vi "Config Save As.vi"(0 "Config Dir":path=path "C:/Users/gtetil/Documents/Projects/TI-cDAQ/Source/Support/Configurations", 1 "Config Extension":string="*.std", 2 "Config Name":string="test.std", 5 "Error IN":errorcluster) -> (14 "Save As":bool, 15 "Config Name OUT":string, 19 "Error OUT":errorcluster)   [LabVIEW 2023]
panel:
  out "Extension":string
  in  "New Config Name:":string caption="Config Name:"
  in  "Cancel Button":bool
  in  "Save As":bool
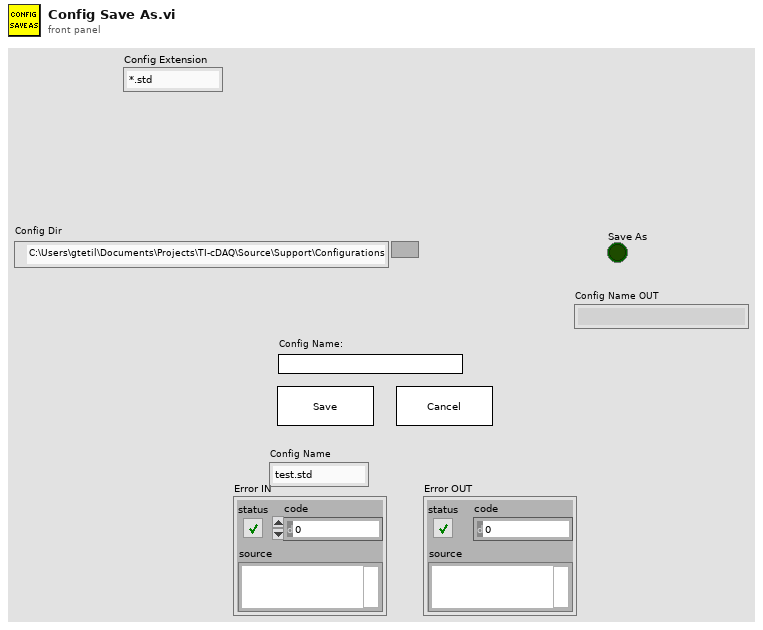
[diagram p1: front panel]
types:
  T1 = cluster{"Error IN":errorcluster, "Config Dir":path, "Config Extension":string, "Save As":bool, "Config Name":string, "Config List":string[]}
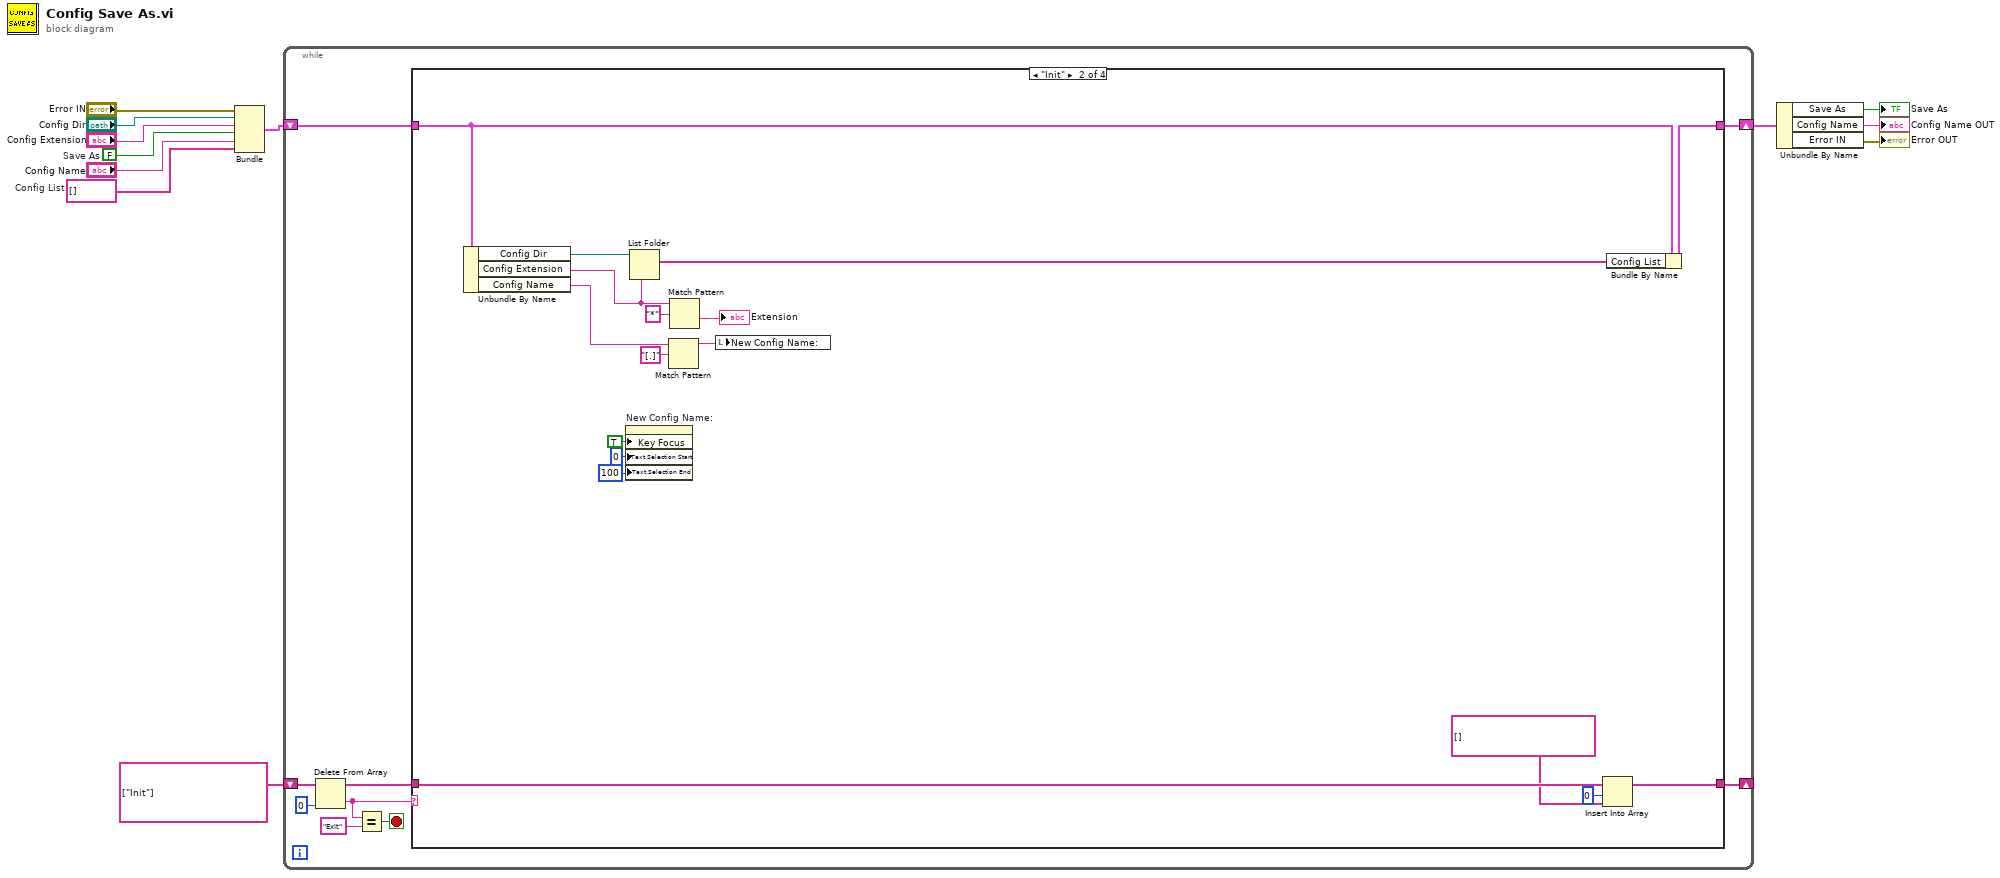
[diagram p0: block diagram]
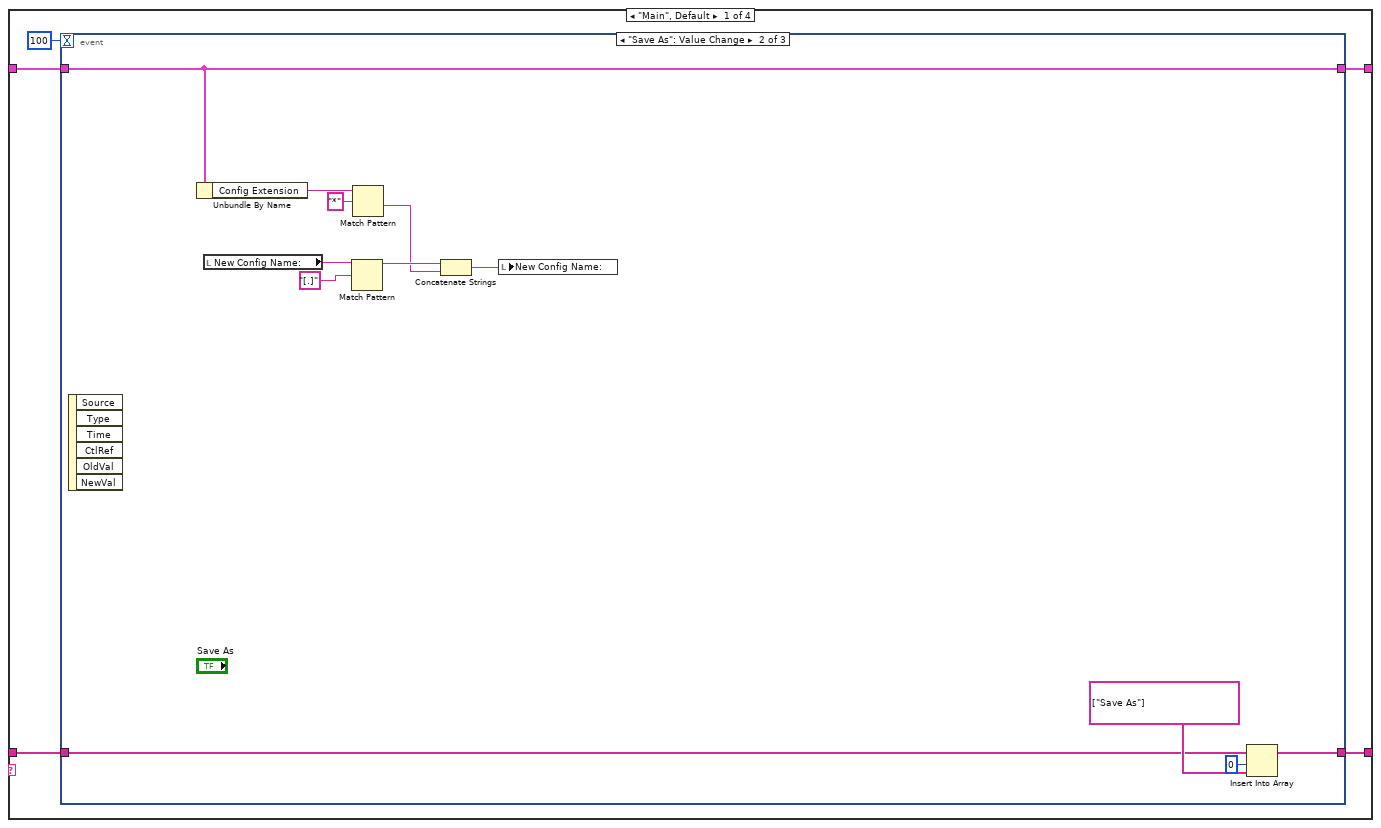
[diagram p2: hidden frame]
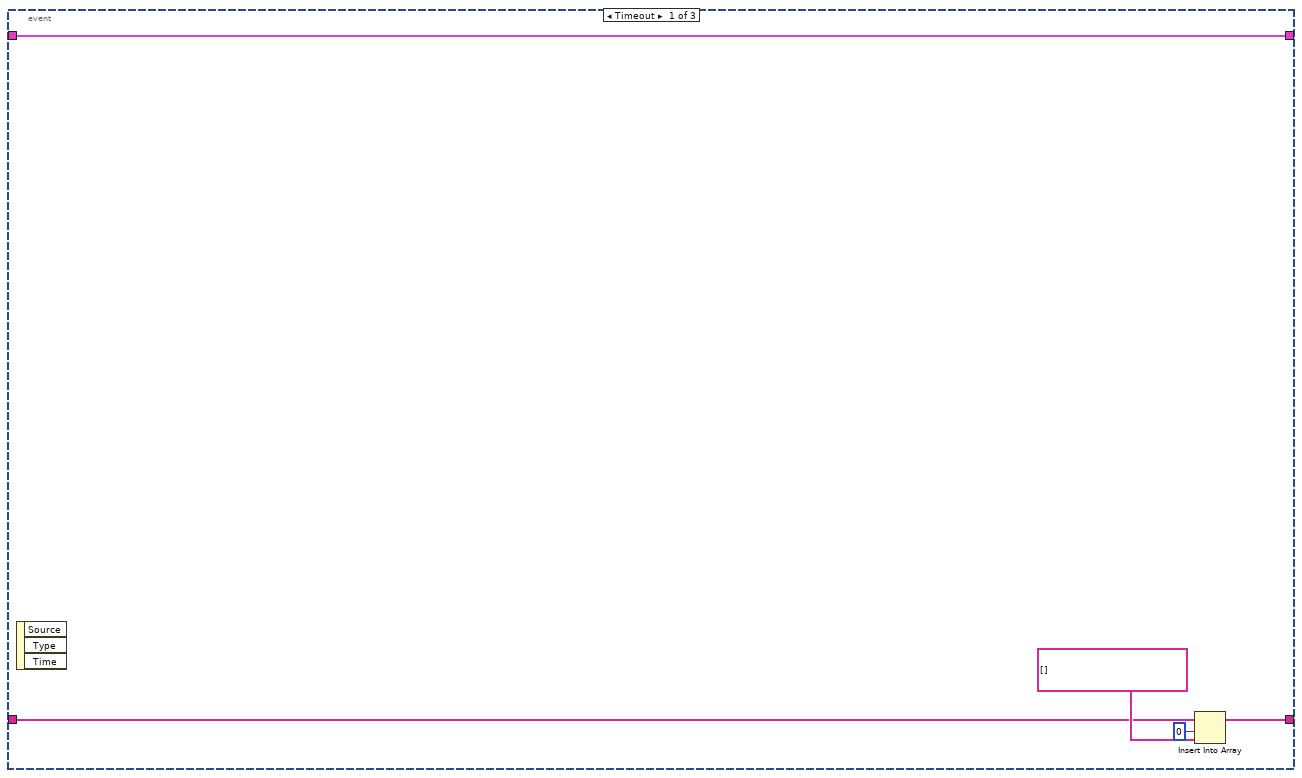
[diagram p3: hidden frame]
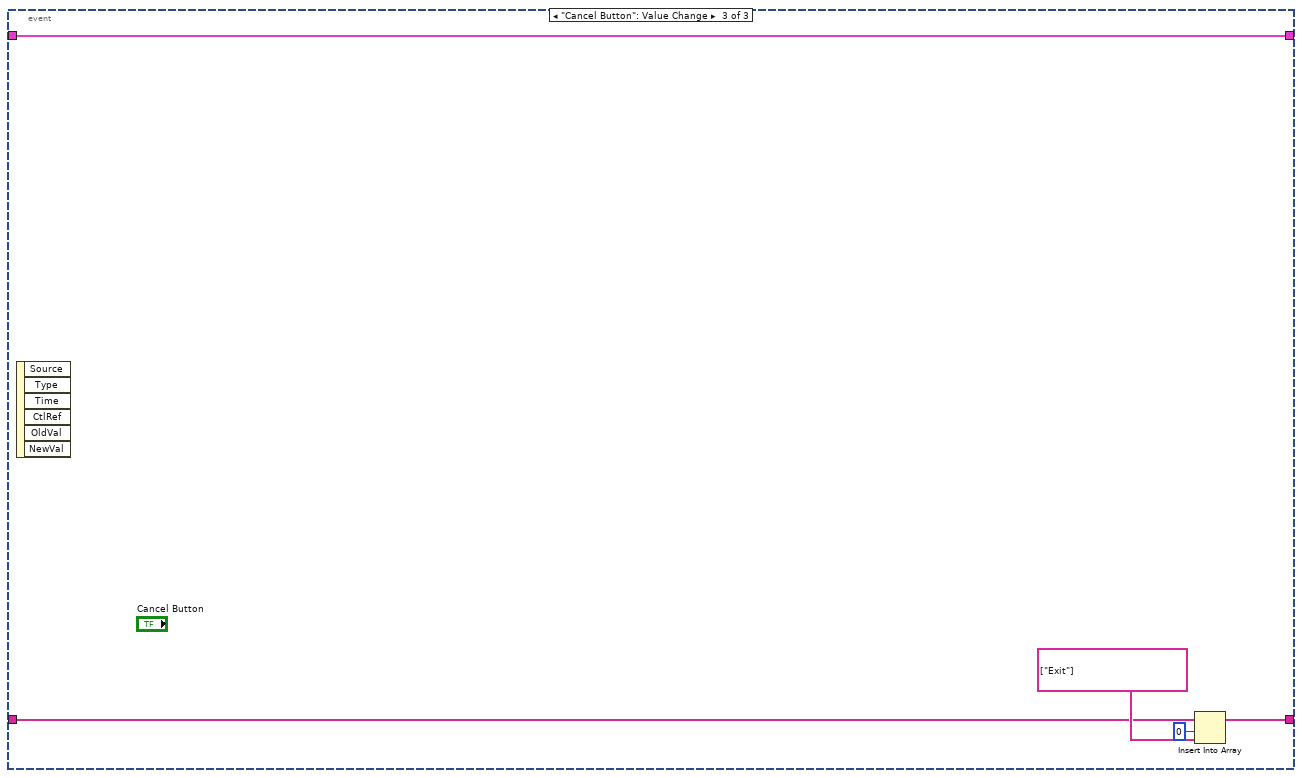
[diagram p4: hidden frame]
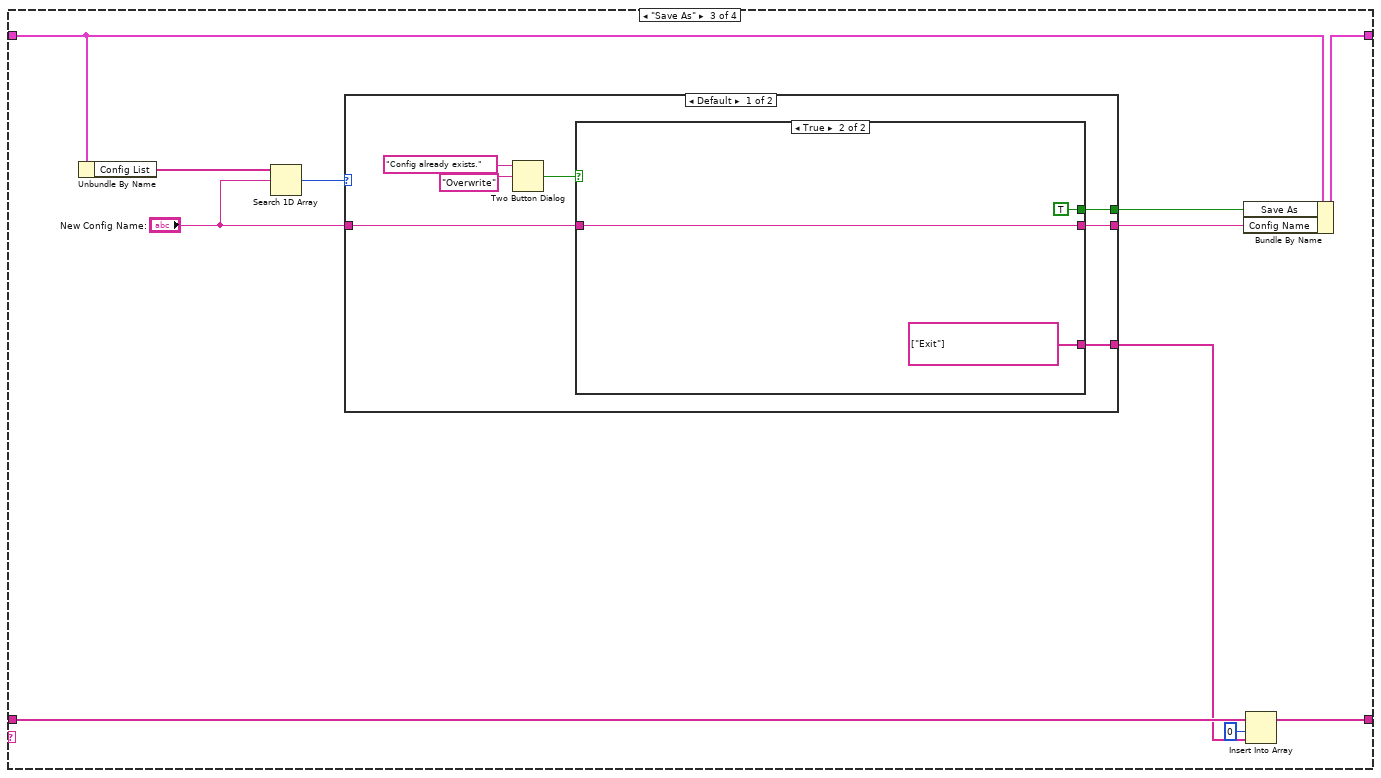
[diagram p5: hidden frame]
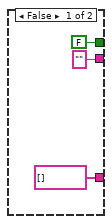
[diagram p6: hidden frame]
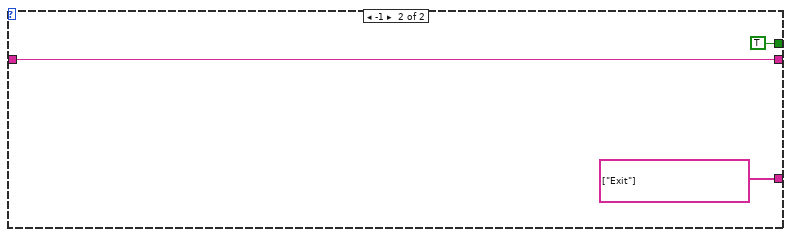
[diagram p7: hidden frame]
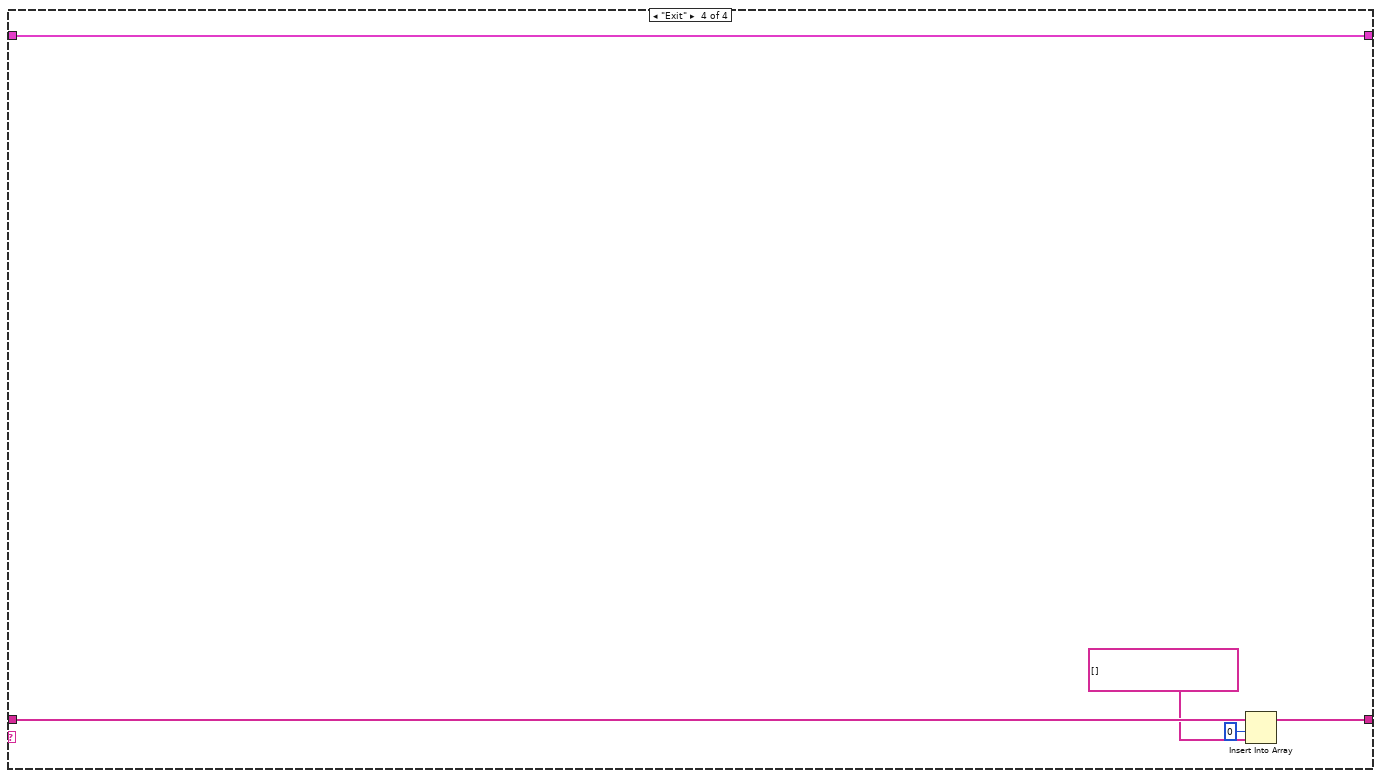
[diagram p8: hidden frame]
diagram:
  w2 = string[] []  # Config List
  w4 = FALSE  # Save As
  n1 = Bundle("Error IN"="Error IN", "Config Dir"="Config Dir", "Config Extension"="Config Extension", "Save As"=w4, "Config Name"="Config Name", "Config List"=w2) -> (w6:T1)  [unwired: 1 in]
  n2 = while {
    shift-right: [w16] -> _
    shift-left: string[] ["Init"] -> [w21]
    shift-right: [w13] -> w9
    shift-left: w6 -> [w14]
    stop <- w17 stop-if-true
    n3 = Delete From Array(array=w21, index=0 ("length")) -> (deleted portion=w18:string, array with subset deleted=w15:string[])  [unwired: 1 in]
    n4 = Equal?(x=w18, y="Exit") -> (x = y?=w17:bool)
    n5 = case shown="\"Init\"" w18 {
      tunnel: [w22 w65 w76 w97] -> w16
      tunnel: w15 -> [w23 w64 w75 w96]
      tunnel: w14 -> [w26 w59 w72 w93]
      tunnel: [w25 w60 w73 w93] -> w13
      frame "Main", Default {
        n6 = event shown="[1] \"Save As\": Value Change" {
          selector: _ -> [_ _ _]
          dyn-events: _ -> [_ _ _]
          timeout: 100 -> [_ _ _]
          tunnel: w26 -> [w31 w39 w44]
          tunnel: [w31 w39 w44] -> w25
          tunnel: w23 -> [w28 w41 w46]
          tunnel: [w27 w40 w45] -> w22
          event Timeout {
            n7 = event-data() -> ()  [unwired: 1 in, 3 out]
            n8 = Insert Into Array(array=w28, index=0, new element=string[] []) -> (w27:string[])
          }
          event "Save As": Value Change {
            n9 = event-data() -> ()  [unwired: 1 in, 6 out]
            n10 = Unbundle By Name(w39) -> ("Config Extension"=w38:string)
            n11 = local read "New Config Name:"() -> (w36:string)
            n12 = Match Pattern(string=w36, regular expression="[.]") -> (before substring=w34:string)  [unwired: 1 in, 3 out]
            n13 = Match Pattern(string=w38, regular expression="*") -> (after substring=w33:string)  [unwired: 1 in, 3 out]
            n14 = Concatenate Strings(w34, w33) -> (w32:string)
            n15 = local write "New Config Name:"(w32) -> ()
            n16 = Insert Into Array(array=w41, index=0, new element=string[] ["Save As"]) -> (w40:string[])
          }
          event "Cancel Button": Value Change {
            n17 = event-data() -> ()  [unwired: 1 in, 6 out]
            n18 = Insert Into Array(array=w46, index=0, new element=string[] ["Exit"]) -> (w45:string[])
          }
        }
      }
      frame "Init" {
        n19 = Unbundle By Name(w59) -> ("Config Dir"=w61:path, "Config Extension"=w53:string, "Config Name"=w56:string)
        n20 = property on="New Config Name:" class="Str"("Key Focus"=TRUE, "Text.Selection Start"=u32 0 ("Text.Selection:Start"), "Text.Selection End"=u32 100 ("Text.Selection:End")) -> ()  [unwired: 2 in, 2 out]
        n21 = List Folder(path=w61, pattern=w53) -> (filenames=w58:string[])  [unwired: 2 in, 3 out]
        n22 = Match Pattern(string=w56, regular expression="[.]") -> (before substring=w55:string)  [unwired: 1 in, 3 out]
        n23 = Match Pattern(string=w53, regular expression="*") -> (after substring=→"Extension":string)  [unwired: 1 in, 3 out]
        n24 = local write "New Config Name:"(w55) -> ()
        n25 = Insert Into Array(array=w64, index=0, new element=string[] []) -> (w65:string[])
        n26 = Bundle By Name(cluster=w59, "Config List"=w58) -> (w60:T1)
      }
      frame "Save As" {
        n27 = Unbundle By Name(w72) -> ("Config List"=w71:string[])
        n28 = Search 1D Array(1D array=w71, element="New Config Name:") -> (index of element=w70:i32)  [unwired: 1 in]
        n29 = case shown="Default" w70 {
          tunnel: [w79 w92] -> w68
          tunnel: "New Config Name:" -> [w78 w92]
          tunnel: [w80 TRUE] -> w67
          tunnel: [w77 string[] ["Exit"]] -> w66
          frame Default {
            n30 = Two Button Dialog(message="Config already exists.", 2:"Overwrite" ("T button name (\"OK\")")) -> (T button?=w81:bool)  [unwired: 1 in]
            n31 = case shown="True" w81 {
              tunnel: [FALSE TRUE] -> w80
              tunnel: ["" ("New Config Name:") w88] -> w79
              tunnel: w78 -> [_ w88]
              tunnel: [string[] [] string[] ["Exit"]] -> w77
              frame False {
              }
              frame True {
              }
            }
          }
          frame -1 {
          }
        }
        n32 = Bundle By Name(cluster=w72, "Save As"=w67, "Config Name"=w68) -> (w73:T1)
        n33 = Insert Into Array(array=w75, index=0, new element=w66) -> (w76:string[])
      }
      frame "Exit" {
        n34 = Insert Into Array(array=w96, index=0, new element=string[] []) -> (w97:string[])
      }
    }
  }
  n35 = Unbundle By Name(w9) -> ("Save As"=→"Save As":bool, "Config Name"=→"Config Name OUT":string, "Error IN"=→"Error OUT":errorcluster)
